vi "InsightCM DataDir Path.vi"() -> (3 "InsightCM Server Path":path)   [LabVIEW 2019, in "Configuration Tool.lvlib"]
uses:
  <vilib>/registry/registry.llb/Registry RtKey.ctl
  <vilib>/registry/registry.llb/Registry SAM.ctl
  <vilib>/registry/registry.llb/Registry View.ctl
  <vilib>/registry/registry.llb/Read Registry Value Simple STR.vi
  Configuration Tool.lvlib
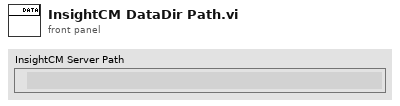
[diagram p1: front panel]
types:
  T1 = typedef "Registry View.ctl" = u16
  T2 = typedef "Registry SAM.ctl" = enum32{"KEY_QUERY_VALUE", "KEY_SET_VALUE", "KEY_CREATE_SUB_KEY", "KEY_ENUMERATE_SUB_KEYS", "KEY_NOTIFY", "KEY_CREATE_LINK", "KEY_READ", "KEY_WRITE", "KEY_ALL_ACCESS", "KEY_READ | KEY_WRITE"}
  T3 = typedef "Registry RtKey.ctl" = enum32{"HKEY_CLASSES_ROOT", "HKEY_CURRENT_USER", "HKEY_LOCAL_MACHINE", "HKEY_USERS", "HKEY_PERFORMANCE_DATA", "HKEY_CURRENT_CONFIG", "HKEY_DYN_DATA"}
  T4 = typedef "Registry refnum.ctl" = refnum<k1>
  T5 = cluster{"numSubKeys":i32, "maxSubKeyLen":i32, "maxSubKeyClassLen":i32}
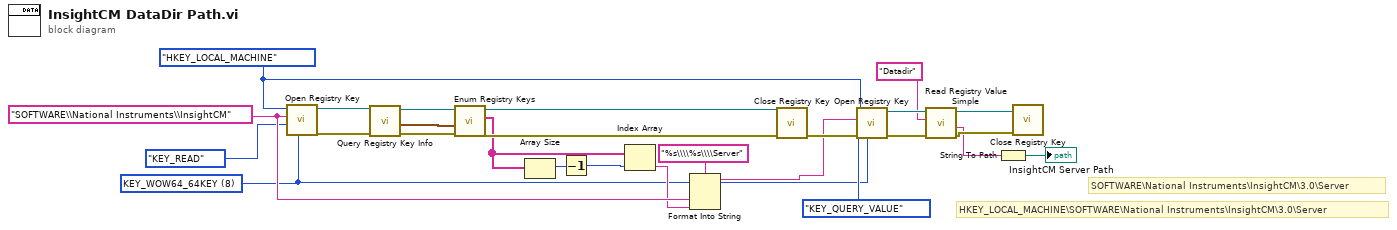
[diagram p0: block diagram]
diagram:
  w7 = T1 8 items=["Default"=0, "KEY_WOW64_64KEY"=8, "KEY_WOW64_32KEY"=9] ("registry view")
  w19 = "SOFTWARE\\National Instruments\\InsightCM" ("subkey")
  w15 = Registry_RtKey."HKEY_LOCAL_MACHINE" ("root key (HKEY_LOCAL_MACHINE)")
  # "SOFTWARE\\National Instruments\\InsightCM\\3.0\\Server"
  # "HKEY_LOCAL_MACHINE\\SOFTWARE\\National Instruments\\InsightCM\\3.0\\Server"
  n1 = call <vilib>:"Open Registry Key.vi"("registry view"=w7, "security access mask (KEY_READ | KEY_WRITE)"=Registry_SAM."KEY_READ", "subkey"=w19, "root key (HKEY_LOCAL_MACHINE)"=w15) -> ("error out"=w25:errorcluster, "refnum out"=w26:T4)  [unwired: 6 in]
  n2 = call <vilib>:"Query Registry Key Info.vi"("error in (no error)"=w25, "refnum"=w26) -> ("error out"=w23:errorcluster, "refnum out"=w24:T4, "subkey info"=w20:T5)  [unwired: 5 in, 2 out]
  n3 = call <vilib>:"Enum Registry Keys.vi"("error in (no error)"=w23, "subkey info"=w20, "refnum"=w24) -> ("error out"=w21:errorcluster, "subkeys"=w4:string[], "refnum out"=w22:T4)  [unwired: 6 in]
  n4 = Array Size(array=w4) -> (size(s)=w3:i32)
  n5 = Decrement(x=w3) -> (x-1=w2:i32)
  n6 = Index Array(array=w4, index=w2) -> (element=w18:string)
  n7 = Format Into String(format string="%s\\\\%s\\\\Server", w19, w18) -> (resulting string=w13:string)  [unwired: 2 in, 1 out]
  n8 = call <vilib>:"Close Registry Key.vi"("error in (no error)"=w21, "refnum"=w22) -> ("error out"=w16:errorcluster)  [unwired: 5 in]
  n9 = call <vilib>:"Open Registry Key.vi"("registry view"=w7, "error in (no error)"=w16, "security access mask (KEY_READ | KEY_WRITE)"=Registry_SAM."KEY_QUERY_VALUE", "subkey"=w13, "root key (HKEY_LOCAL_MACHINE)"=w15) -> ("error out"=w11:errorcluster, "refnum out"=w12:T4)  [unwired: 5 in]
  n10 = call-poly <vilib>:"Read Registry Value Simple.vi"("error in (no error)"=w11, "value"="Datadir", "refnum"=w12) -> ("error out"=w9:errorcluster, "String/Binary data"=w6:string, "refnum out"=w10:T4)  [unwired: 3 in, 1 out]
  n11 = String To Path(string=w6) -> (path=→"InsightCM Server Path":path)
  n12 = call <vilib>:"Close Registry Key.vi"("error in (no error)"=w9, "refnum"=w10) -> ()  [unwired: 5 in, 1 out]
